vi "Alarm Settings.vi"(8 "error in (no error)":errorcluster, 11 "Alarm Settings in":T1) -> (0 "error out":errorcluster, 2 "Modified":bool, 3 "Alarm Settings out":T1)   [LabVIEW 2021]
uses:
  Alarm Threholds.ctl
  Alarm Settings Data.ctl
panel:
  in  "Exit":bool=TRUE
  in  "Cancel":bool
  in  "Save":bool
  in  "LL":dbl
  in  "L":dbl
  in  "H":dbl
  in  "HH":dbl
  # "Alarm Settings"
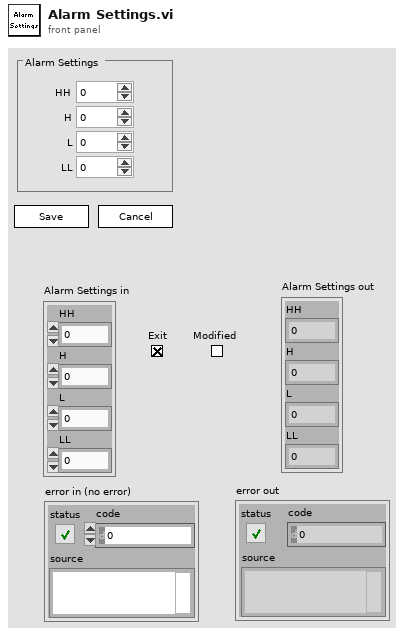
[diagram p1: front panel]
types:
  T1 = typedef "Alarm Threholds.ctl" = cluster{"HH":dbl, "H":dbl, "L":dbl, "LL":dbl}
  T2 = typedef "Alarm Settings Data.ctl" = cluster{"Alarm Thresholds":T1, "Modified":bool}
  T3 = enum32{"Invalid", "Standard", "Closed", "Hidden", "Minimized", "Maximized"}
  T4 = enum8{"Enabled", "Disabled", "Disabled and Grayed Out"}
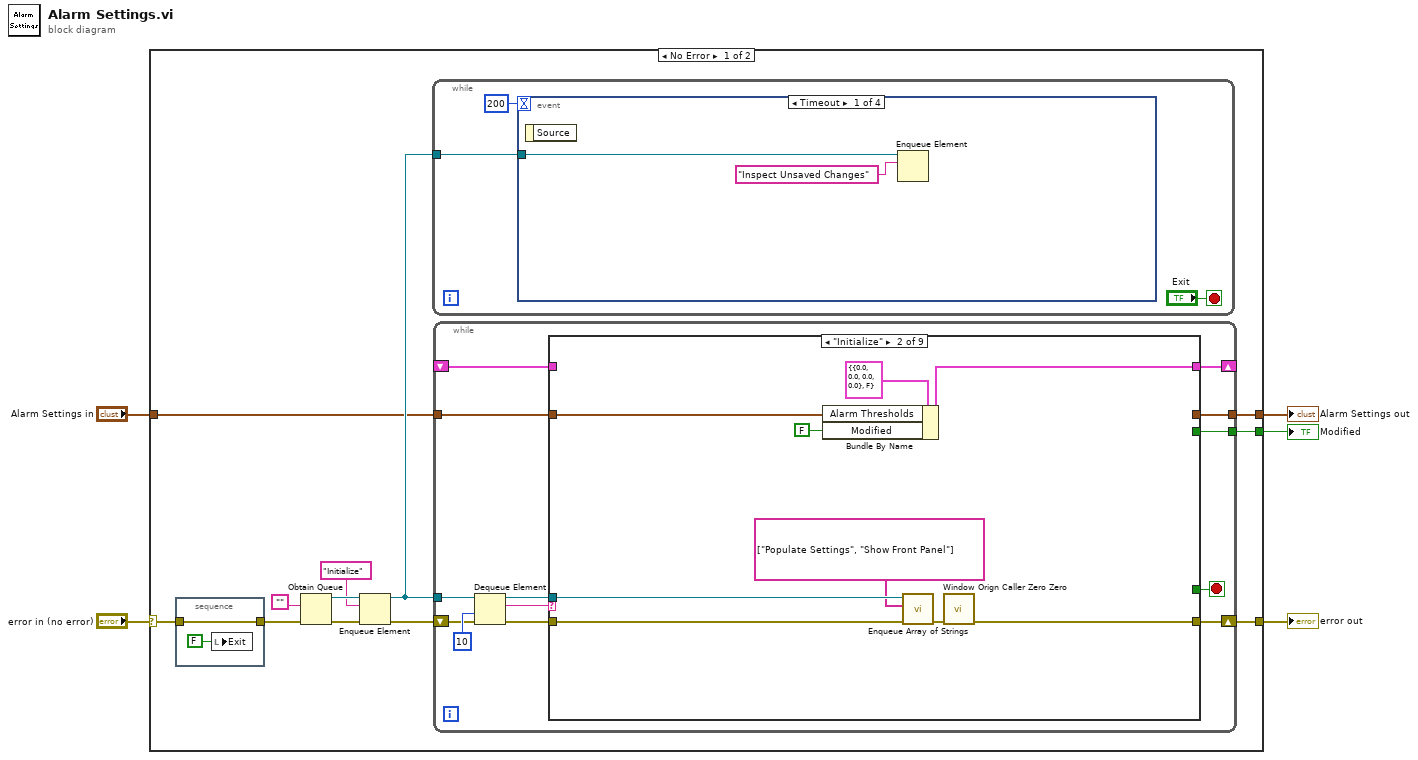
[diagram p0: block diagram]
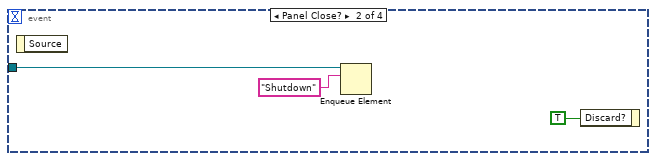
[diagram p2: hidden frame]
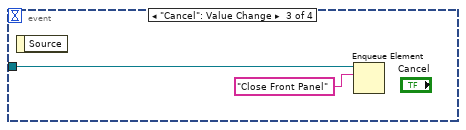
[diagram p3: hidden frame]
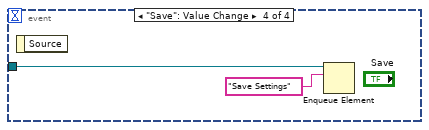
[diagram p4: hidden frame]
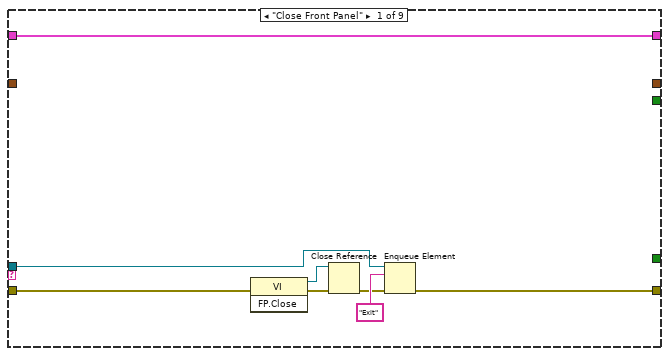
[diagram p5: hidden frame]
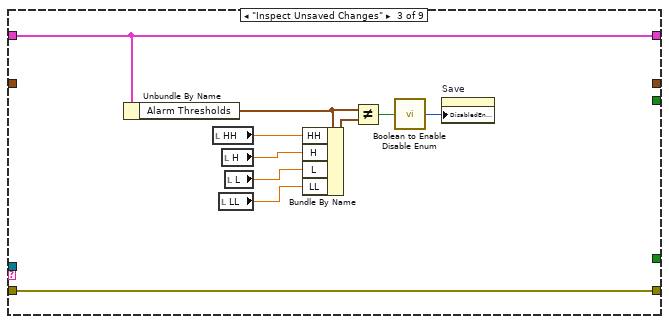
[diagram p6: hidden frame]
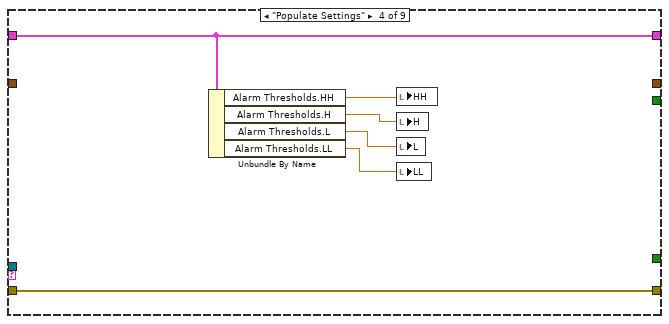
[diagram p7: hidden frame]
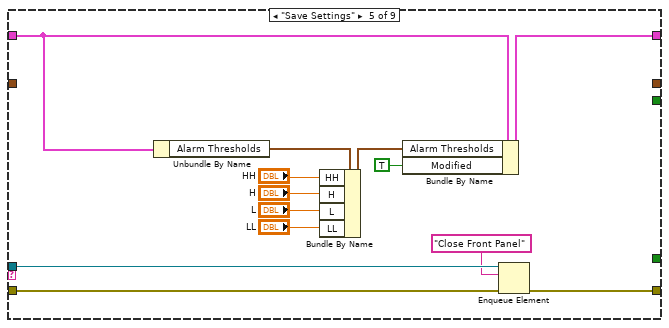
[diagram p8: hidden frame]
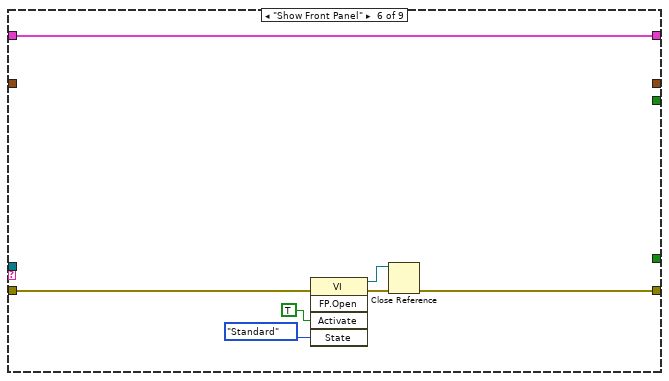
[diagram p9: hidden frame]
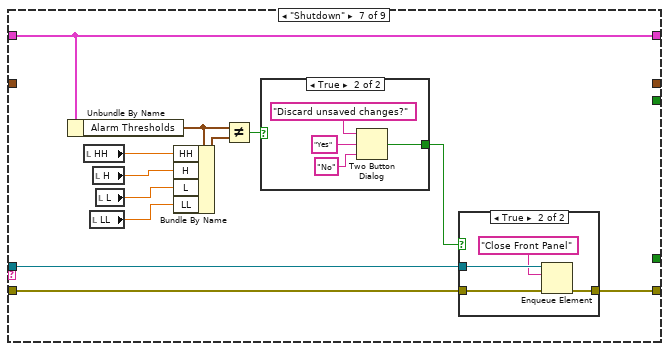
[diagram p10: hidden frame]
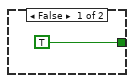
[diagram p12: hidden frame]
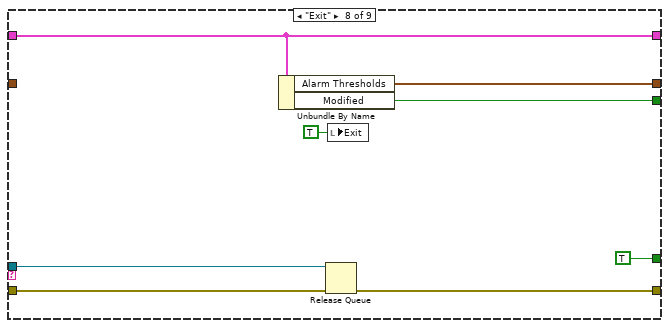
[diagram p13: hidden frame]
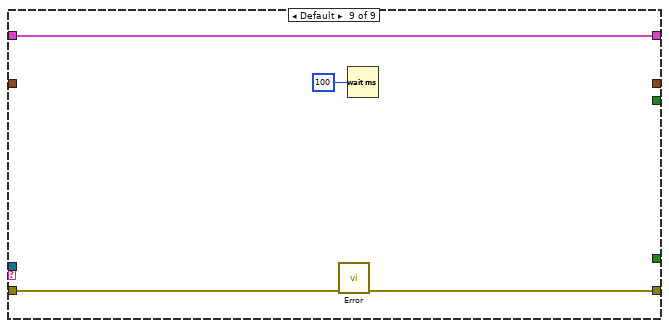
[diagram p14: hidden frame]
diagram:
  n1 = case shown="No Error" "error in (no error)" {
    selector: "error in (no error)" -> [w10 w133]
    tunnel: [w9 w133] -> w4
    tunnel: [w8 _] -> w3
    tunnel: [w7 w132] -> w2
    tunnel: "Alarm Settings in" -> [w6 w132]
    frame No Error {
      n2 = stacked-sequence {
        tunnel: w10 -> [w18]
        tunnel: [w18] -> w11
        frame #0 {
          n3 = local write "Exit"(FALSE ("Exit")) -> ()
        }
      }
      n4 = Obtain Queue(element data type="", error in (no error)=w11) -> (queue out=w16:refnum<queue>, error out=w17:errorcluster)  [unwired: 3 in, 1 out]
      n5 = Enqueue Element(queue=w16, element="Initialize", error in (no error)=w17) -> (queue out=w12:refnum<queue>, error out=w13:errorcluster)  [unwired: 1 in, 1 out]
      n6 = while {
        tunnel: w12 -> [w21]
        stop <- "Exit" stop-if-true
        n7 = event shown="[0] Timeout" {
          selector: _ -> [_ _ _ _]
          dyn-events: _ -> [_ _ _ _]
          timeout: 200 -> [_ _ _ _]
          tunnel: w21 -> [w23 w26 w28 w30]
          event Timeout {
            n8 = event-data() -> ()  [unwired: 1 in, 1 out]
            n9 = Enqueue Element(queue=w23, element="Inspect Unsaved Changes" ("Queue Element")) -> ()  [unwired: 2 in, 3 out]
          }
          event Panel Close? {
            n10 = event-data() -> ()  [unwired: 1 in, 1 out]
            n11 = Enqueue Element(queue=w26, element="Shutdown" ("Queue Element")) -> ()  [unwired: 2 in, 3 out]
            n12 = event-data("Discard?"=TRUE) -> ()  [unwired: 1 in, 1 out]
          }
          event "Cancel": Value Change {
            n13 = event-data() -> ()  [unwired: 1 in, 1 out]
            n14 = Enqueue Element(queue=w28, element="Close Front Panel" ("Queue Element")) -> ()  [unwired: 2 in, 3 out]
          }
          event "Save": Value Change {
            n15 = event-data() -> ()  [unwired: 1 in, 1 out]
            n16 = Enqueue Element(queue=w30, element="Save Settings" ("Queue Element")) -> ()  [unwired: 2 in, 3 out]
          }
        }
      }
      n17 = while {
        tunnel: w12 -> [w40]
        shift-left: w13 -> [w39]
        shift-right: [w44] -> w9
        shift-right: [w42] -> _
        shift-left: _ -> [w43]
        tunnel: [w34] -> w8
        tunnel: [w33] -> w7
        tunnel: w6 -> [w32]
        stop <- w35 stop-if-true
        n18 = Dequeue Element(queue=w40, timeout in ms (-1)=10, error in (no error)=w39) -> (queue out=w36:refnum<queue>, element=w37:string, error out=w38:errorcluster)  [unwired: 1 out]
        n19 = case shown="\"Initialize\"" w37 {
          tunnel: w38 -> [w49 w54 w71 w77 w79 w92 w107 w127 w129]
          tunnel: [w46 w58 w71 w77 w84 w91 w108 w125 w128] -> w44
          tunnel: w36 -> [w45 w56 _ _ w88 _ w106 w126 _]
          tunnel: w43 -> [w52 _ w67 w76 w90 w97 w99 w124 w130]
          tunnel: [w52 w60 w67 w76 w89 w97 w99 w124 w130] -> w42
          tunnel: [_ _ _ _ _ _ _ TRUE _] -> w35
          tunnel: [_ _ _ _ _ _ _ w121 _] -> w34
          tunnel: [_ _ _ _ _ _ _ w120 _] -> w33
          tunnel: w32 -> [_ w57 _ _ _ _ _ _ _]
          frame "Close Front Panel" {
            n20 = invoke class="VI" method="FP.Close"(error in=w49) -> (reference out=w50:refnum<vi>, error out=w51:errorcluster)  [unwired: 2 in, 1 out]
            n21 = Close Reference(reference=w50, error in (no error)=w51) -> (error out=w47:errorcluster)
            n22 = Enqueue Element(queue=w45, element="Exit", error in (no error)=w47) -> (error out=w46:errorcluster)  [unwired: 1 in, 2 out]
          }
          frame "Initialize" {
            n23 = Bundle By Name(cluster=T2 {"Alarm Thresholds"={"HH"=0.0, "H"=0.0, "L"=0.0, "LL"=0.0}, "Modified"=FALSE} ("Edit Module State Data"), "Alarm Thresholds"=w57, "Modified"=FALSE) -> (w60:T2)
            n24 = call "Enqueue Array of Strings.vi"("error in (no error)"=w54, "Array"=string[] ["Populate Settings", "Show Front Panel"] ("Array of EventNames"), "queue"=w56) -> ("error out"=w53:errorcluster)  [unwired: 7 in, 1 out]
            n25 = call "Window Orign Caller Zero Zero.vi"("error in (no error)"=w53) -> ("error out"=w58:errorcluster)  [unwired: 14 in]
          }
          frame "Inspect Unsaved Changes" {
            n26 = Unbundle By Name(w67) -> ("Alarm Thresholds"=w69:T1)
            n27 = local read "HH"() -> (w66:dbl)
            n28 = local read "LL"() -> (w63:dbl)
            n29 = local read "H"() -> (w65:dbl)
            n30 = local read "L"() -> (w64:dbl)
            n31 = Bundle By Name(cluster=w69, "HH"=w66, "H"=w65, "L"=w64, "LL"=w63) -> (w70:T1)
            n32 = Not Equal?(x=w69, y=w70) -> (x != y?=w68:bool)
            n33 = call "Boolean to Enable Disable Enum.vi"("Enable"=w68) -> ("State"=w62:T4)
            n34 = property on="Save" class="Bool"("DisabledEnum"=w62) -> ()  [unwired: 2 in, 2 out]
          }
          frame "Populate Settings" {
            n35 = Unbundle By Name(w76) -> ("Alarm Thresholds.HH"=w75:dbl, "Alarm Thresholds.H"=w74:dbl, "Alarm Thresholds.L"=w73:dbl, "Alarm Thresholds.LL"=w72:dbl)
            n36 = local write "HH"(w75) -> ()
            n37 = local write "H"(w74) -> ()
            n38 = local write "L"(w73) -> ()
            n39 = local write "LL"(w72) -> ()
          }
          frame "Save Settings" {
            n40 = Unbundle By Name(w90) -> ("Alarm Thresholds"=w87:T1)
            n41 = Bundle By Name(cluster=w87, "HH"="HH", "H"="H", "L"="L", "LL"="LL") -> (w78:T1)
            n42 = Bundle By Name(cluster=w90, "Alarm Thresholds"=w78, "Modified"=TRUE ("Canceled")) -> (w89:T2)
            n43 = Enqueue Element(queue=w88, element="Close Front Panel", error in (no error)=w79) -> (error out=w84:errorcluster)  [unwired: 1 in, 2 out]
          }
          frame "Show Front Panel" {
            n44 = invoke class="VI" method="FP.Open"(error in=w92, "Activate"=TRUE ("Activate?"), "State"=T3."Standard") -> (reference out=w93:refnum<vi>, error out=w94:errorcluster)  [unwired: 2 in, 3 out]
            n45 = Close Reference(reference=w93, error in (no error)=w94) -> (error out=w91:errorcluster)
          }
          frame "Shutdown" {
            n46 = Unbundle By Name(w99) -> ("Alarm Thresholds"=w104:T1)
            n47 = local read "HH"() -> (w103:dbl)
            n48 = local read "LL"() -> (w100:dbl)
            n49 = local read "H"() -> (w102:dbl)
            n50 = local read "L"() -> (w101:dbl)
            n51 = Bundle By Name(cluster=w104, "HH"=w103, "H"=w102, "L"=w101, "LL"=w100) -> (w105:T1)
            n52 = Not Equal?(x=w104, y=w105) -> (x != y?=w98:bool)
            n53 = case shown="True" w98 {
              tunnel: [TRUE ("T button?") w116] -> w109
              frame False {
              }
              frame True {
                n54 = Two Button Dialog(message="Discard unsaved changes?", 1:"No" ("F button name (\"Cancel\")"), 2:"Yes" ("T button name (\"OK\")")) -> (T button?=w116:bool)
              }
            }
            n55 = case shown="True" w109 {
              tunnel: w107 -> [w110 w114]
              tunnel: w106 -> [_ w113]
              tunnel: [w110 w112] -> w108
              frame False {
              }
              frame True {
                n56 = Enqueue Element(queue=w113, element="Close Front Panel", error in (no error)=w114) -> (error out=w112:errorcluster)  [unwired: 1 in, 2 out]
              }
            }
          }
          frame "Exit" {
            n57 = Unbundle By Name(w124) -> ("Alarm Thresholds"=w120:T1, "Modified"=w121:bool)
            n58 = Release Queue(queue=w126, error in (no error)=w127) -> (error out=w125:errorcluster)  [unwired: 1 in, 2 out]
            n59 = local write "Exit"(TRUE ("Exit")) -> ()
          }
          frame Default {
            n60 = call "Error.vi"("error in (no error)"=w129) -> ("error out"=w128:errorcluster)  [unwired: 13 in, 1 out]
            n61 = Wait (ms)(milliseconds to wait=u32 100) -> ()  [unwired: 1 out]
          }
        }
      }
    }
    frame Error {
    }
  }
  "error out" <- w4
  "Alarm Settings out" <- w2
  "Modified" <- w3
